vi "array dinension - 1D template.vi"() -> ()   [LabVIEW 2018]
panel:
  out "Array Size":i32
  in  "Index":i32
  in  "Array":dbl[](array[numeric])
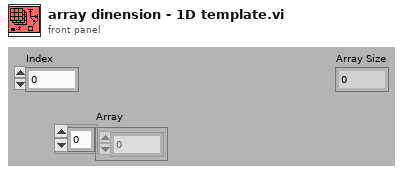
[diagram p1: front panel]
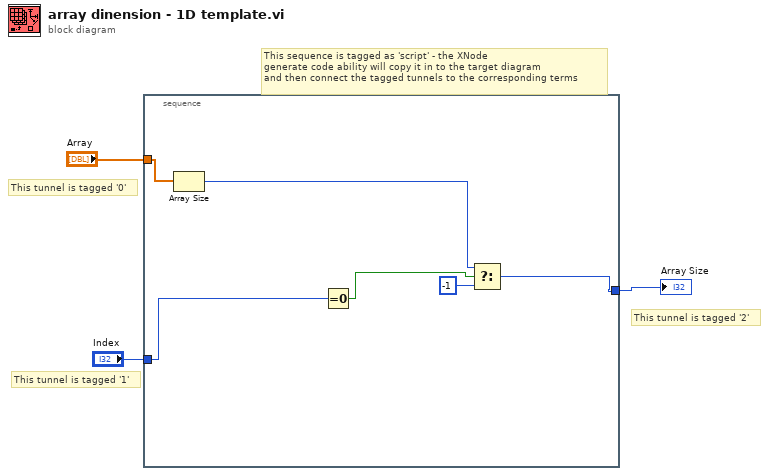
[diagram p0: block diagram]
diagram:
  # "This tunnel is tagged '2'"
  # "This tunnel is tagged '1'"
  # "This tunnel is tagged '0'"
  # "This sequence is tagged as 'script' - the XNode \ngenerate code ability will copy it in to the target diagram\nand then connect the tagged tunnels to the corresponding terms"
  n1 = stacked-sequence {
    tunnel: "Array" -> [w7]
    tunnel: "Index" -> [w5]
    tunnel: [w8] -> w1
    frame #0 {
      n2 = Array Size(array=w7) -> (size(s)=w6:i32)
      n3 = Equal To 0?(x=w5) -> (x = 0?=w4:bool)
      n4 = Select(t=w6, s=w4, f=-1) -> (s? t:f=w8:i32)
    }
  }
  "Array Size" <- w1
